vi "Set Server Key File.vi"(10 "Server Key File (.key)":path, 11 "OOP Server in":refnum<class "HVC6.lvclass">) -> (3 "OOP Server out":refnum<class "HVC6.lvclass">)   [LabVIEW 2019, in "HVC6.lvlib" / "HVC6.lvclass"]
uses:
  HVC6.lvclass
  HVC6.lvclass/HVC6.ctl
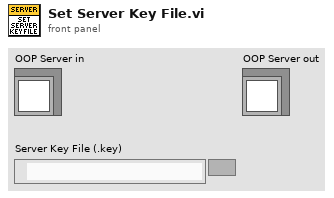
[diagram p1: front panel]
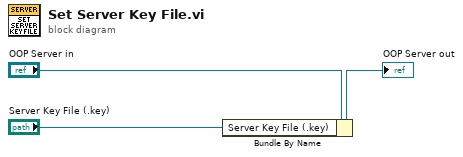
[diagram p0: block diagram]
diagram:
  n1 = Bundle By Name(cluster="OOP Server in", "Server Key File (.key)"="Server Key File (.key)") -> (→"OOP Server out":refnum<class "HVC6.lvclass">)
